vi "ARM_ACQUIRE.vi"(8 "error in":errorcluster) -> (0 "error out":errorcluster)   [LabVIEW 2023]
uses:
  <vilib>/Rock Robotics/WPI/ThirdParty/JAS_Junk/TrajLib/Conv_Deg_Radians.vi
  ARM_GLOBALS.vi
  <vilib>/Rock Robotics/WPI/ThirdParty/Phoenix-LabVIEW/CANCoder/Get/CTRE_Phoenix_CANcoder_GetSensorData.vi
  <vilib>/Rock Robotics/WPI/ThirdParty/JAS_Junk/TrajLib/Trajectory_Library.lvlib
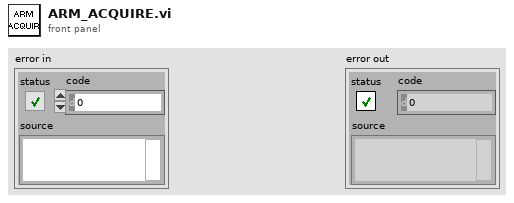
[diagram p1: front panel]
types:
  T1 = typedef "CTRE_Phoenix_CANcoder_DeviceRef.ctl" = cluster{"DeviceStatus":errorcluster, "Device Number":u8, "Handle":u64, "UsageFrame":u32, "Library Path":path}
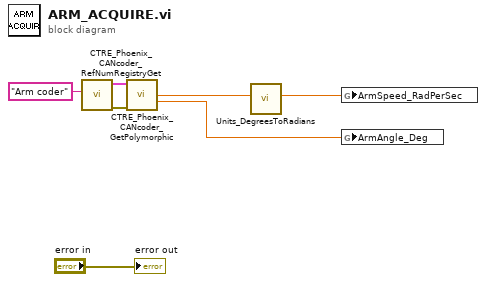
[diagram p0: block diagram]
diagram:
  n1 = call <vilib>:"CTRE_Phoenix_CANcoder_RefNumRegistryGet.vi"("refnum name"="Arm coder") -> ("error out"=w5:errorcluster, "CTRE_CANcoder_DeviceRef"=w6:T1)  [unwired: 9 in]
  n2 = call-poly <vilib>:"CTRE_Phoenix_CANcoder_GetPolymorphic.vi"("CTRE_CANcoder_DeviceRef"=w6, "error in"=w5) -> ("Velocity"=w2:dbl, "Absolute Position"=w4:dbl)  [unwired: 9 in, 3 out]
  n3 = call <vilib>:"Units_DegreesToRadians.vi"("Degrees"=w2) -> ("Radians"=w1:dbl)  [unwired: 10 in]
  n4 = global write "ARM_GLOBALS.vi" "ArmSpeed_RadPerSec"(w1) -> ()
  n5 = global write "ARM_GLOBALS.vi" "ArmAngle_Deg"(w4) -> ()
  "error out" <- "error in"
